vi "VoltageGeneratorWithDMM.vi"() -> ()   [LabVIEW 2023]
panel:
  out "Most Recent Measurement":dbl
  out "Plot":dynamicdata(graph)
  in  "Measurement Type":enum16{"Voltage", "Current", "Resistance"}(ring)
  in  "Power":bool
  in  "Voltage Control":dbl(knob) scale=-10.0..10.0
  out "Output Voltage":dbl(knob) scale=-10.0..10.0
  in  "Output Enable":bool
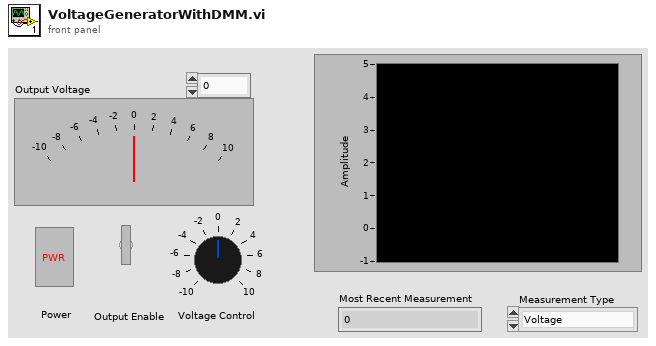
[diagram p1: front panel]
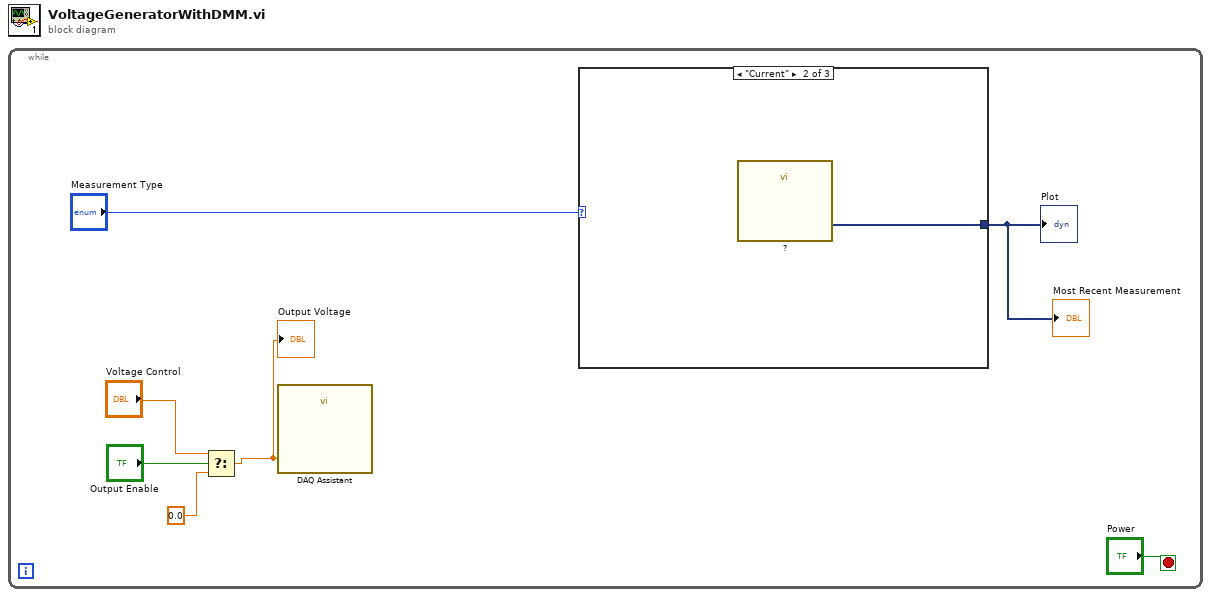
[diagram p0: block diagram]
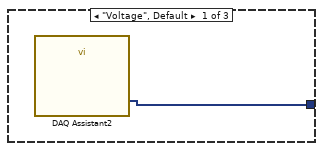
[diagram p2: hidden frame]
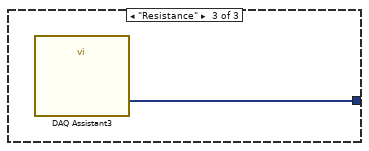
[diagram p3: hidden frame]
diagram:
  n1 = while {
    stop <- "Power" stop-if-true
    n2 = Select(t="Voltage Control", s="Output Enable", f=0.0) -> (s? t:f=w3:dbl)
    "Output Voltage" <- w3
    n3 = call "DAQ Assistant"("data"=w3) -> ()  [unwired: 17 in, 2 out]
    n4 = case shown="\"Current\"" "Measurement Type" {
      tunnel: [w8 w9 w10] -> w1
      frame "Voltage", Default {
        n5 = call "DAQ Assistant2"() -> ("data"=w8:dynamicdata)  [unwired: 17 in, 2 out]
      }
      frame "Current" {
        n6 = call "?"() -> ("data"=w9:dynamicdata)  [unwired: 17 in, 2 out]
      }
      frame "Resistance" {
        n7 = call "DAQ Assistant3"() -> ("data"=w10:dynamicdata)  [unwired: 17 in, 2 out]
      }
    }
    "Plot" <- w1
    "Most Recent Measurement" <- w1
  }
